vi "ConvertMac.vi"(8 "error in (no error)":errorcluster, 11 "Mac (with or without semicolons)":string) -> (0 "error out":errorcluster, 2 "Mac without semi":string, 3 "Mac with semi":string)   [LabVIEW 2013]
uses:
  Test Globals/Global 1.vi
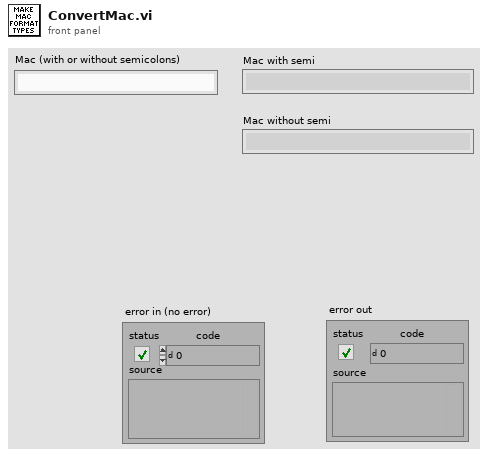
[diagram p1: front panel]
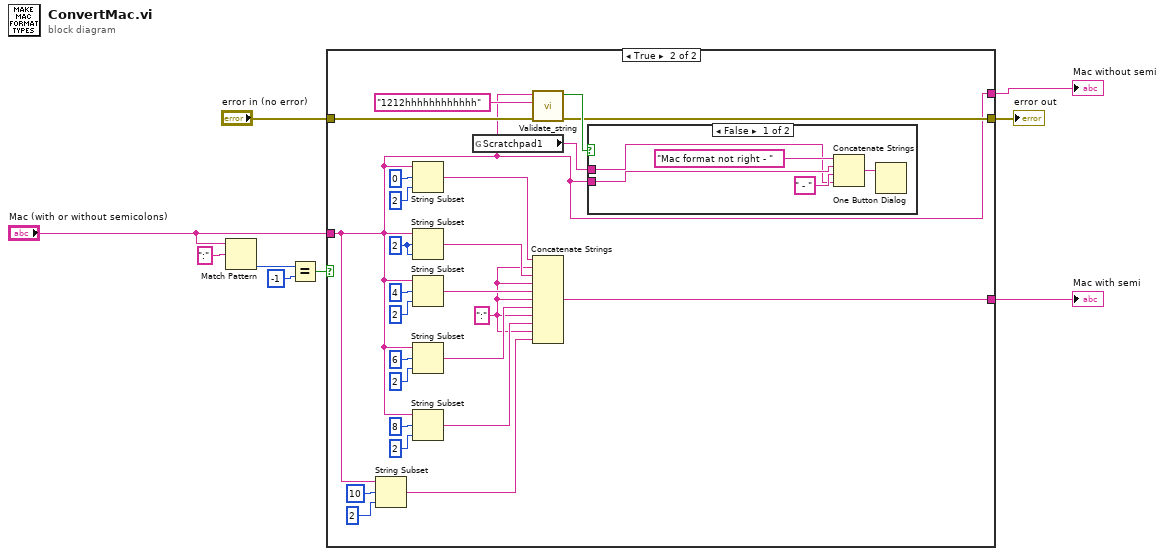
[diagram p0: block diagram]
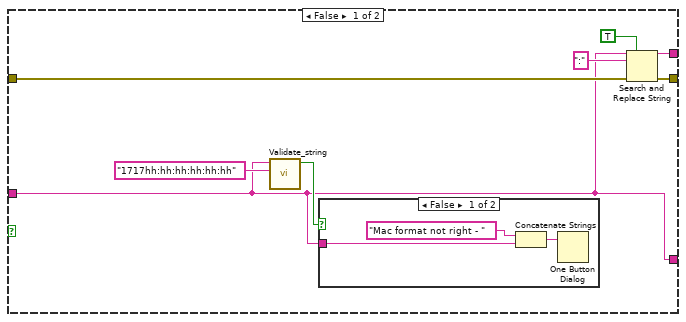
[diagram p2: hidden frame]
diagram:
  n1 = Match Pattern(string="Mac (with or without semicolons)", regular expression=":") -> (offset past match=w8:i32)  [unwired: 1 in, 3 out]
  n2 = Equal?(x=w8, y=-1) -> (x = y?=w6:bool)
  n3 = case shown="True" w6 {
    tunnel: "Mac (with or without semicolons)" -> [w10 w22]
    tunnel: "error in (no error)" -> [w16 w24]
    tunnel: [w15 w23] -> w3
    tunnel: [w13 w22] -> w2
    tunnel: [w10 w27] -> w1
    frame False {
      n4 = call "Validate_string.vi"("String data format"="1717hh:hh:hh:hh:hh:hh", "String"=w10) -> ("String Valid"=w12:bool)  [unwired: 8 in, 1 out]
      n5 = case shown="False" w12 {
        tunnel: w10 -> [w18 _]
        frame False {
          n6 = Concatenate Strings("Mac format not right - " ("message"), w18) -> (w20:string)
          n7 = One Button Dialog(message=w20) -> ()  [unwired: 1 in, 1 out]
        }
        frame True {
        }
      }
      n8 = Search and Replace String(replace all?=TRUE ("replace all? (F)"), input string=w10, search string=":", error in=w16) -> (result string=w13:string, error out=w15:errorcluster)  [unwired: 4 in, 2 out]
    }
    frame True {
      w29 = ":" ("string")
      w44 = 2 ("offset (0)")
      n9 = String Subset(string=w22, offset (0)=10, length (rest)=2 ("length (rest)")) -> (substring=w28:string)
      n10 = String Subset(string=w22, offset (0)=0, length (rest)=2 ("length (rest)")) -> (substring=w34:string)
      n11 = String Subset(string=w22, offset (0)=w44, length (rest)=w44) -> (substring=w33:string)
      n12 = String Subset(string=w22, offset (0)=4, length (rest)=2 ("length (rest)")) -> (substring=w32:string)
      n13 = String Subset(string=w22, offset (0)=6, length (rest)=2 ("length (rest)")) -> (substring=w31:string)
      n14 = String Subset(string=w22, offset (0)=8, length (rest)=2 ("length (rest)")) -> (substring=w30:string)
      n15 = global read "Global 1.vi" "Scratchpad1"() -> (w21:string)
      n16 = call "Validate_string.vi"("error in (no error)"=w24, "String data format"="1212hhhhhhhhhhhh", "String"=w22) -> ("error out"=w23:errorcluster, "String Valid"=w25:bool)  [unwired: 7 in]
      n17 = Concatenate Strings(w34, w29, w33, w29, w32, w29, w31, w29, w30, w29, w28) -> (w27:string)
      n18 = case shown="False" w25 {
        tunnel: w22 -> [w48 _]
        tunnel: w21 -> [w46 _]
        frame False {
          n19 = Concatenate Strings("Mac format not right - " ("message"), w48, " - " ("string"), w46) -> (w50:string)
          n20 = One Button Dialog(message=w50) -> ()  [unwired: 1 in, 1 out]
        }
        frame True {
        }
      }
    }
  }
  "error out" <- w3
  "Mac without semi" <- w2
  "Mac with semi" <- w1
